vi "Eye Params.vi"() -> ()   [LabVIEW 2010]
panel:
  in  "Eye Params":dbl[](array[numeric])
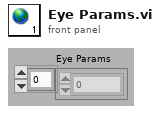
[diagram p1: front panel]
diagram:
